vi "créer code EMBALLAGE_PAGO_V2.0.vi"(0 "DIVISION":enum16{"FLATPROP", "MEDIC"}(ring), 1 "N° carton":u8=1, 2 "DATA cmde":T2={"n°article FAS"="12-216C-04521 EQIFIL 417mA 14.4ohm", "n° cmde FAS"="03838/08-01.07.01", "quantité cmde"="75", "ID LIG cmde"="966584", "n° cmde client"="CF-08-0253/2", "nom client"="EMS Electro Medical System", "n° article client"="EL-360", "indice revision client"="03", "société de facturation"="Fas medic", "langue a utiliser"="FR"}, 5 "article":string="12-216C-04521 EQIFIL 417mA 14.4ohm", 7 "Nb pièces par carton":u8=25, 9 "Tableau n° valves":string[](array[string])=["112105740008010001", "112105740008010002", "112105740008010003", "112105740008010004", "112105740008010005", "112105740008010006", "112105740008010007", "112105740008010008", "112105740008010009", "112105740008010010", "112105740008010011", "112105740008010012", "112105740008010013", "112105740008010014", "112105740008010015", "112105740008010016", "112105740008010017", "112105740008010018", "112105740008010019", "112105740008010020", "112105740008010022", "112105740008010030", "112105740008010099", "112105740008020006", "112105740008020066"], 11 "error in (no error)":errorcluster caption="entrée d'erreur (pas d'erreur)", 12 "Tableau \nlots OUT":string[][](array[string]), 13 "Paramètres Produit (PP)":T1={"Numéro T121"="", "Créateur"="", "Date de création"="", "Date de modification"="", "indice produit"="", "Code Barre fixe"="", "Affiche n° Client [Oui/Non]"="", "Fichier PTV"="", "Nbr de valves / Cartons"="", "Mélange des lots posiible [Oui/Non] "="", "Affiche code barre client [Oui/Non]"="Non", "Fichier PP valve sur embase"="", "Valve Direct/Compensée [D/C]"="D"} caption="Paramètres produit", 14 "affiche code bar client":string="non") -> (6 "chaine  à écrire":string="ZB\nUS\nq600\nD7\nN\nR150,20\nI8,12,001\rA0,40,0,2,1,1,N,\"Carton : 1/2\"\rA0,85,0,2,1,1,N,\"Nb de valves : 25\"\rA0,130,0,2,1,1,N,\"Nø valves :\"\rA144,130,0,1,1,1,N,\"04235698, 05050505, 06060606, 06125478\"\rA144,146,0,1,1,1,N,\"06235511, 07070707, 08023326, 08080808\"\rA144,162,0,1,1,1,N,\"08080808, 08090909, 08110030, 08112347\"\rA144,178,0,1,1,1,N,\"08120003, 08120004, 08120025, 08121114\"\rA144,194,0,1,1,1,N,\"08123625, 08141254, 08152365, 08235644\"\rA144,210,0,1,1,1,N,\"08336251, 08452145, 08521456, 09040006\"\rA144,226,0,1,1,1,N,\"09090909\"\rB64,260,0,1,1,20,56,N,\"12-216C-04520 EQIFIL 104mA 36ohm\"\rA58,324,0,3,1,1,N,\"12...", 15 "error out":errorcluster caption="sortie d'erreur")   [LabVIEW 2020]
uses:
  Flatprop/Flatprop - Standard/XML/Control/PP Param_3.ctl
panel:
  out "n° cmde client":string="1/1"
  out "Destinataire":string="1/1"
  out "n° commande FAS":string="03838/08-07.01.01"
  out "n° valves 9-12":string
  out "Ref client":string="EL-360 "
  out "nom sous code bar client":string="EL-360  03 08010802 7"
  out "n° valves 46-50":string
  out "n° valves 41-45":string
  out "n° valves 36-40":string
  out "n° valves 25-28":string
  out "n° valves 21-24":string
  out "n° valves 17-20":string
  out "n° valves 13-16":string
  out "n° valves 5-8":string="08020006, 08020066"
  out "n° valves 1-4":string="08010003, 08010006, 08010009, 08010022, 08010099"
  out "Quantité":string="7/100"
  out "carton":string="1/1"
  out "nom valve FAS":string="12-216C-04520 EQIFIL 104mA 36ohm"
  # "Destinataire:"
  # "N°commande :"
  # "Quantité:"
  # "Votre ref.:"
  # "N° valves :\n(P/N)"
  # "FASmedic s.a.\nZone industrielle\nCH-1607 Palézieux-Gare\nTél.+41(0)21 907 79 71\nwww.fasmedic.com"
  # "N°article FAS:"
  # "N°commande FAS:"
  # "Carton :"
  # "etiquette"
  # "(Lien interchangeable)"
  # "emballage"
  # "emballage"
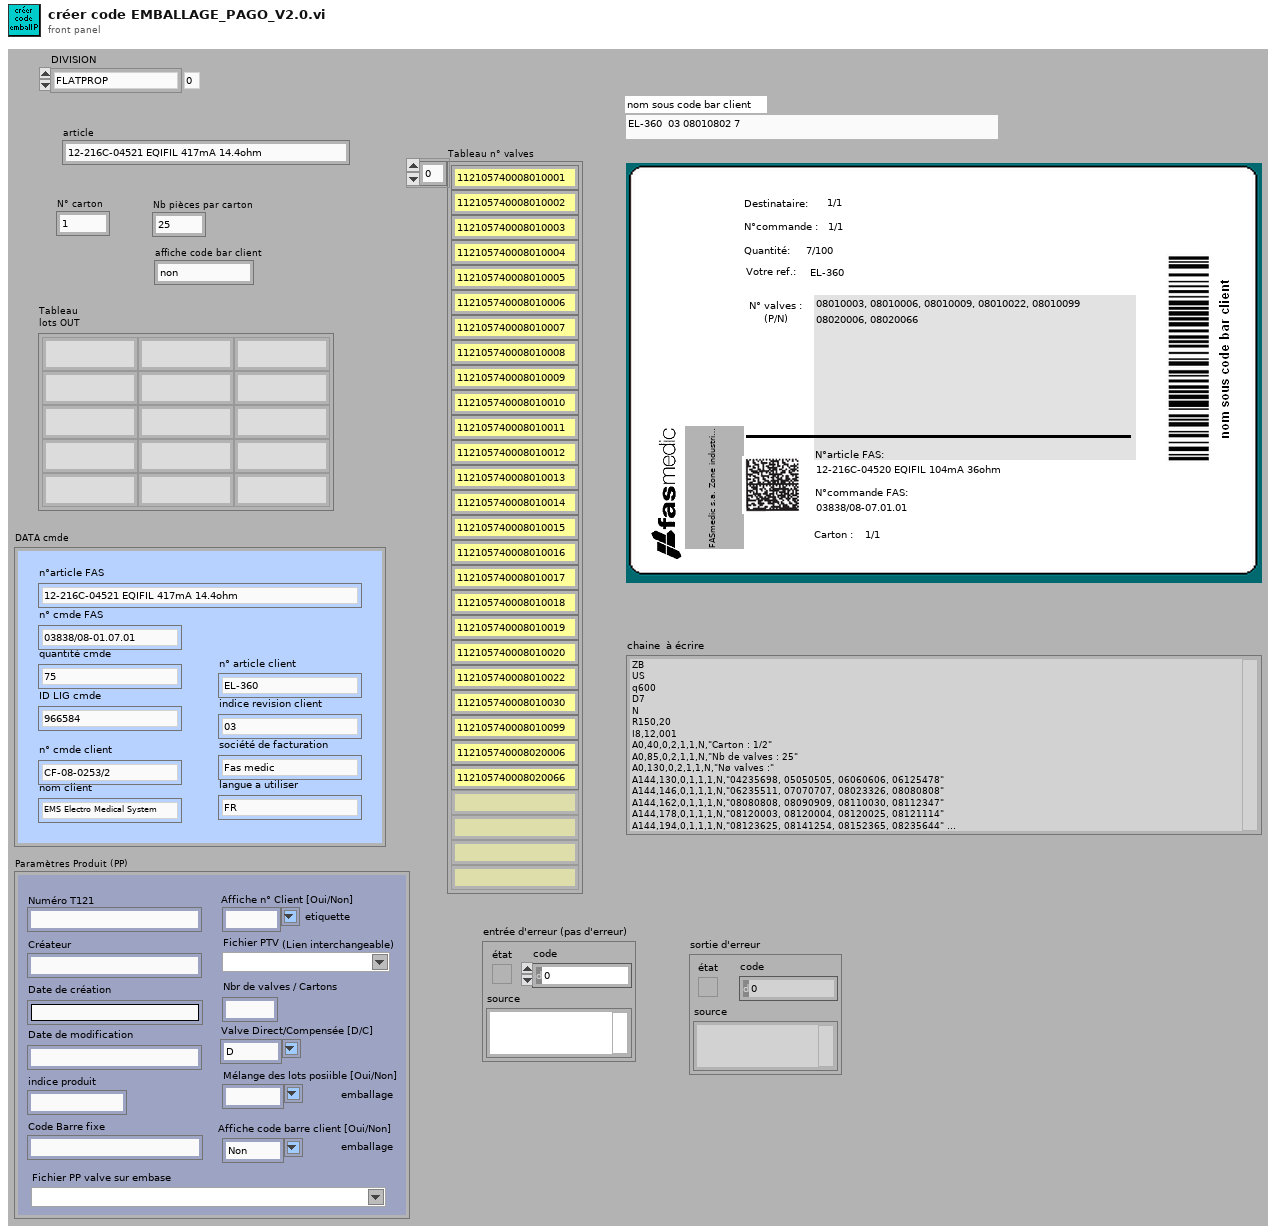
[diagram p1: front panel]
types:
  T1 = typedef "PP Param_3.ctl" = cluster{"Numéro T121":string, "Créateur":string, "Date de création":string, "Date de modification":string, "indice produit":string, "Code Barre fixe":string, "Affiche n° Client [Oui/Non]":string, "Fichier PTV":string, "Nbr de valves / Cartons":string, "Mélange des lots posiible [Oui/Non] ":string, "Affiche code barre client [Oui/Non]":string, "Fichier PP valve sur embase":string, "Valve Direct/Compensée [D/C]":string}
  T2 = typedef "DATA commande.ctl" = cluster{"n°article FAS":string, "n° cmde FAS":string, "quantité cmde":string, "ID LIG cmde":string, "n° cmde client":string, "nom client":string, "n° article client":string, "indice revision client":string, "société de facturation":string, "langue a utiliser":string}
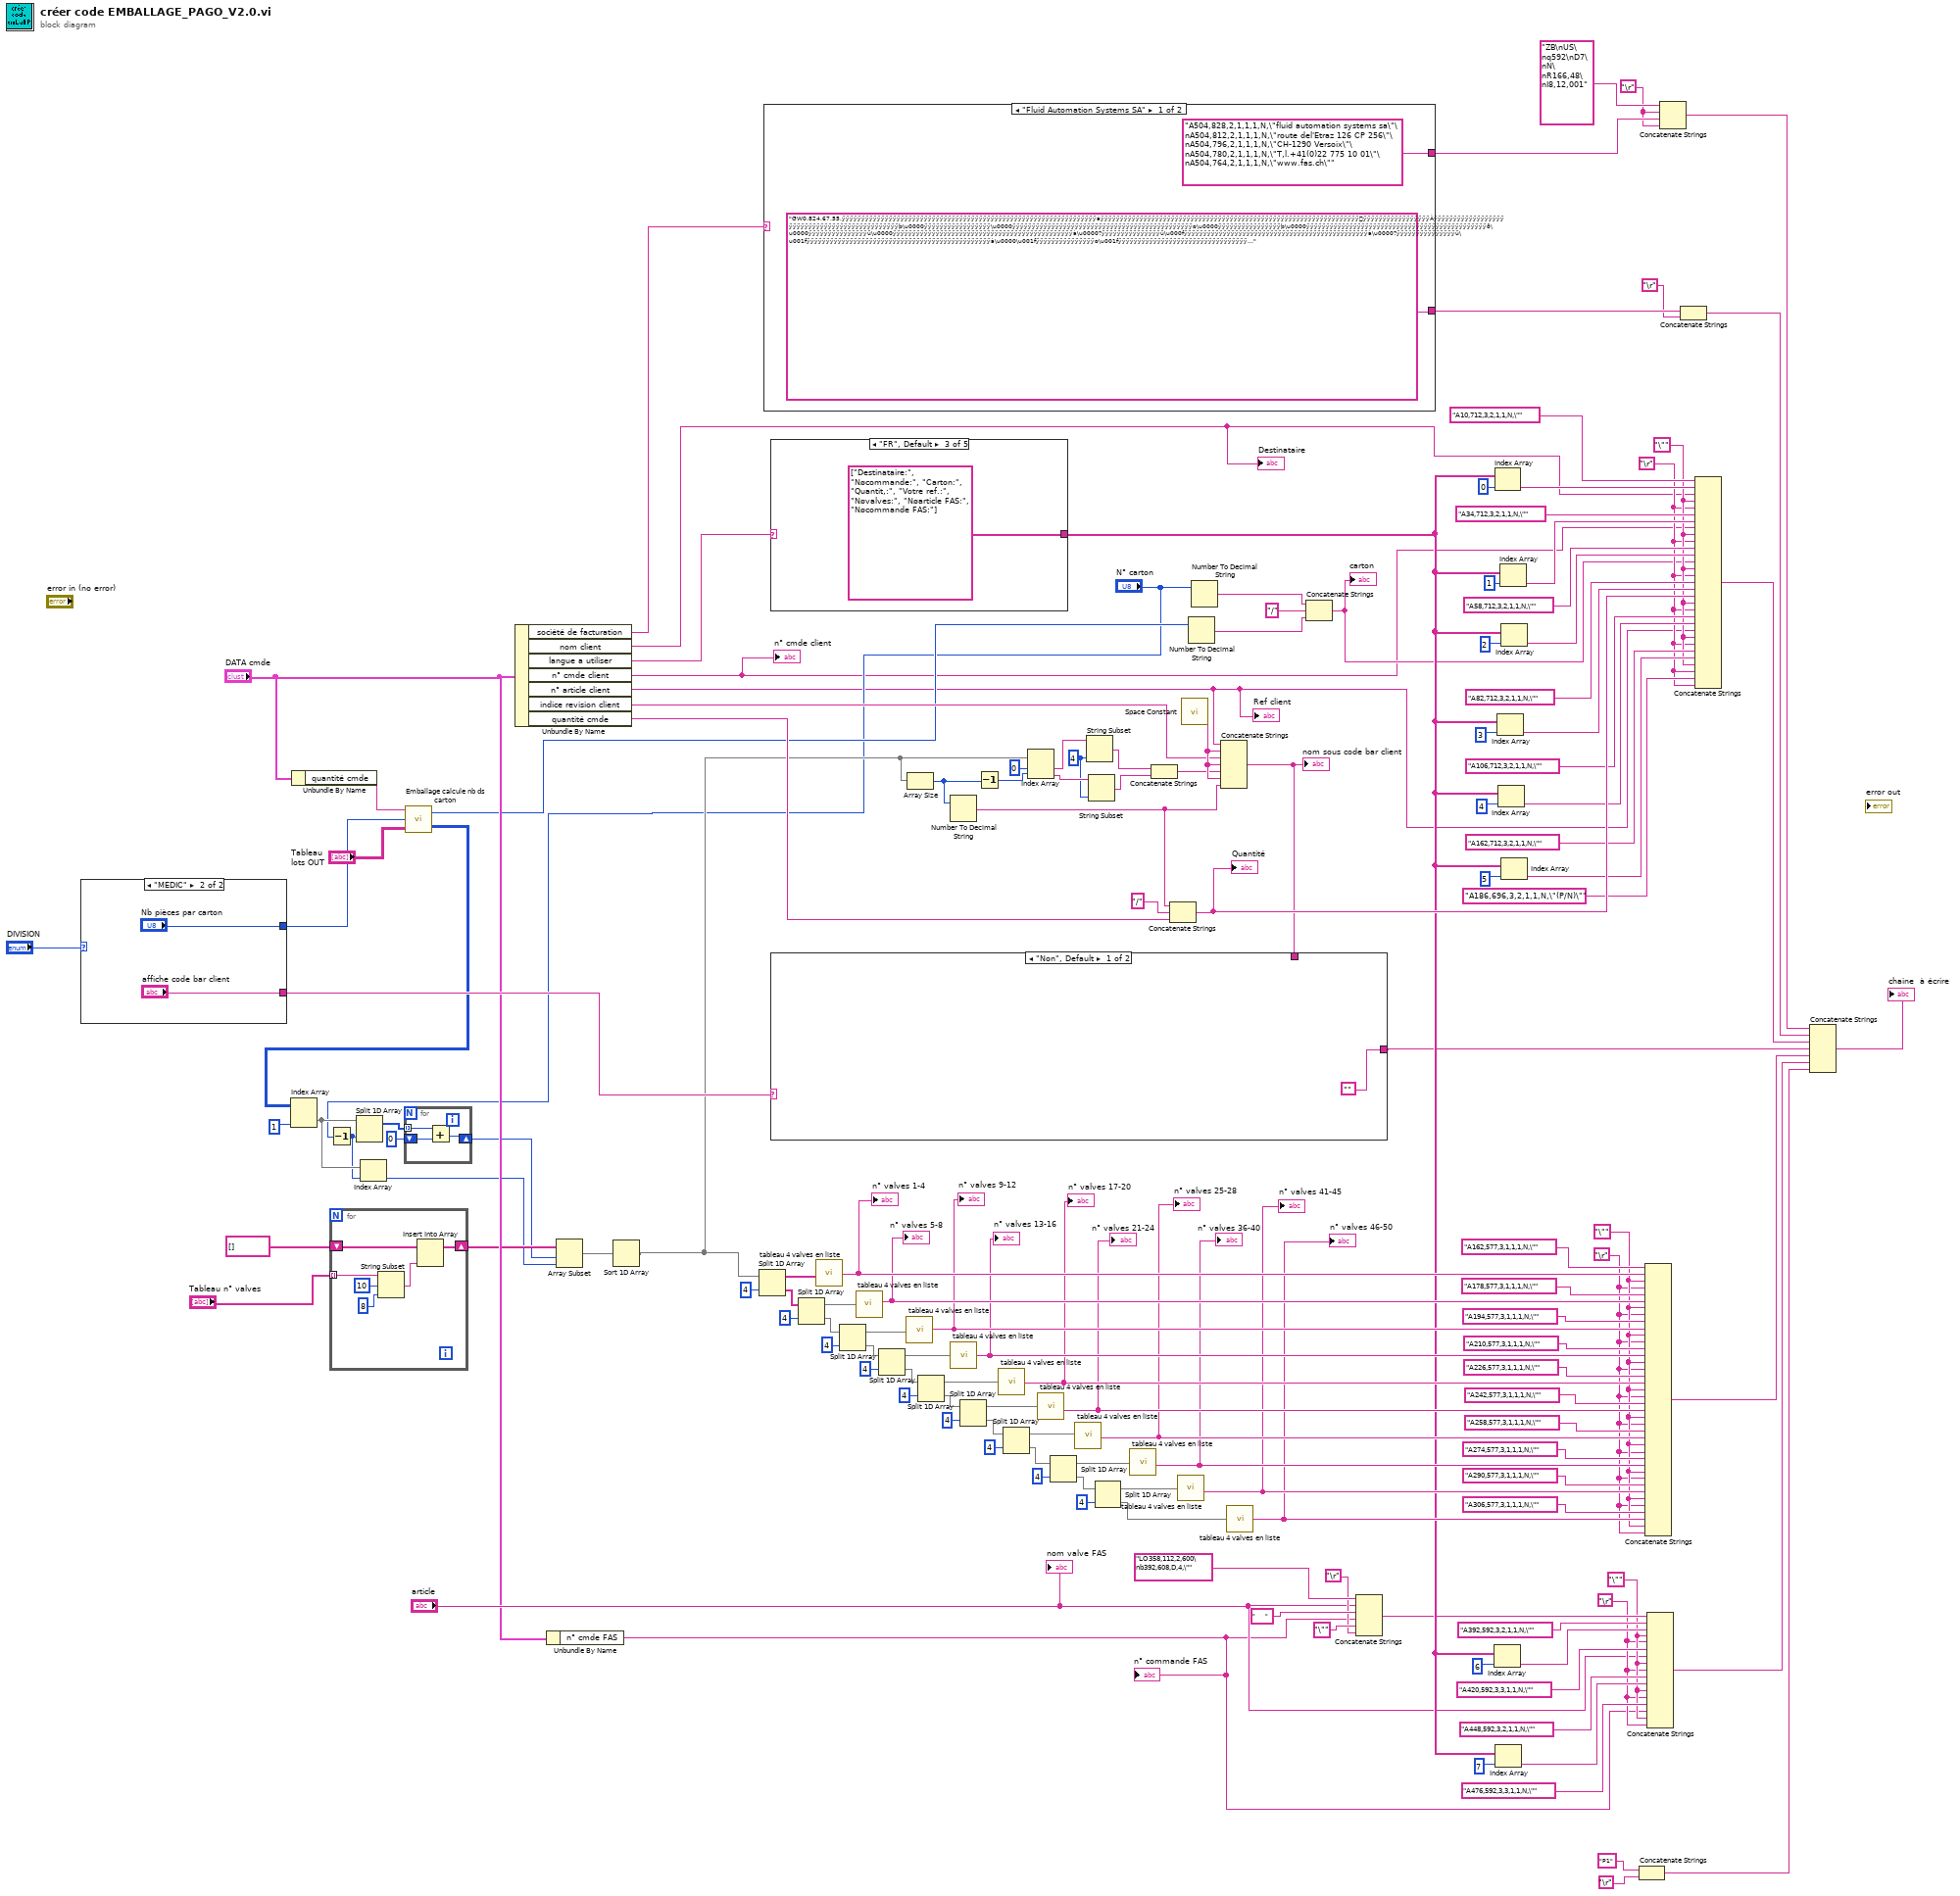
[diagram p0: block diagram]
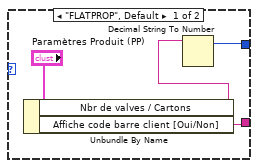
[diagram p2: hidden frame]
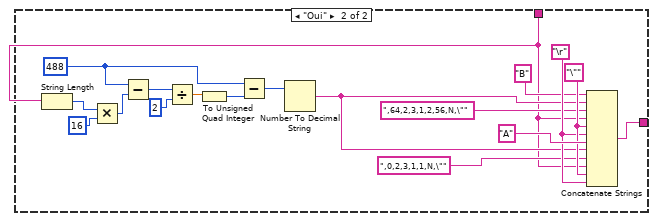
[diagram p3: hidden frame]
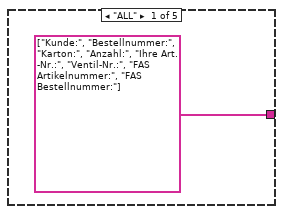
[diagram p4: hidden frame]
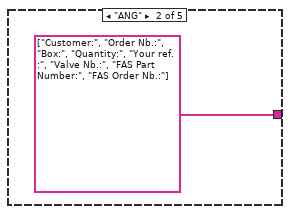
[diagram p5: hidden frame]
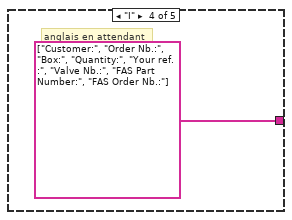
[diagram p6: hidden frame]
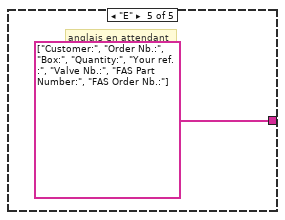
[diagram p7: hidden frame]
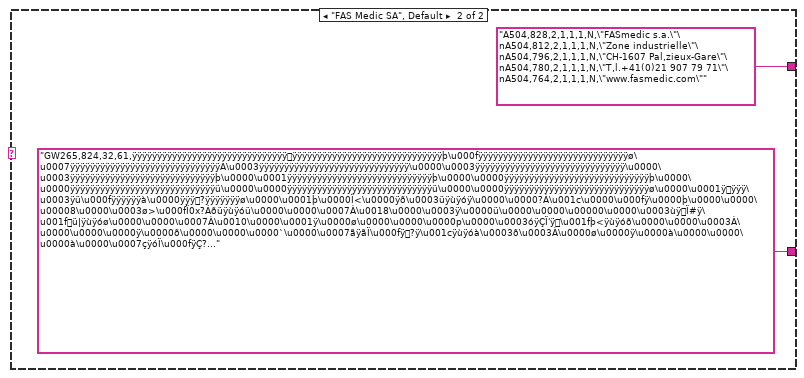
[diagram p8: hidden frame]
diagram:
  w47 = "\r"
  w48 = "\""
  w64 = "\""
  w63 = "\r"
  w87 = "\""
  w85 = "\r"
  w107 = "\r"
  w116 = 4 ("longueur (reste)")
  n1 = case shown="\"MEDIC\"" "DIVISION" {
    tunnel: [w149 "affiche code bar client"] -> w28
    tunnel: [w151 "Nb pièces par carton"] -> w25
    frame "FLATPROP", Default {
      n2 = Unbundle By Name("Paramètres Produit (PP)") -> ("Nbr de valves / Cartons"=w150:string, "Affiche code barre client [Oui/Non]"=w149:string)
      n3 = Decimal String To Number(string=w150) -> (offset past number=w151:i32)  [unwired: 2 in, 1 out]
    }
    frame "MEDIC" {
    }
  }
  n4 = Unbundle By Name("DATA cmde") -> ("quantité cmde"=w23:string)
  n5 = Decrement(x="N° carton") -> (x-1=w12:u8)
  n6 = for {
    tunnel: "Tableau n° valves" -> [w160] mode=indexing
    shift-right: [w157] -> w18
    shift-left: string[] [] -> [w156]
    n7 = String Subset(string=w160, offset (0)=10, length (rest)=8 ("longueur (reste)")) -> (substring=w158:string)
    n8 = Insert Into Array(array=w156, new element=w158) -> (w157:string[])  [unwired: 1 in]
  }
  n9 = call "Emballage calcule nb ds carton.vi"("Tableau \nlots OUT"="Tableau \nlots OUT", 3:w25, "Quantité de la cmde"=w23) -> ("Tab n° carton - nb ds carton"=w7:i32[][], "Nb total cartons"=w6:i32)
  n10 = Index Array(array=w7, index (col)=1 ("indice désactivé (col)")) -> (element=w13:i32[])  [unwired: 1 in]
  n11 = Split 1D Array(array=w13, index=w12) -> (first subarray=w15:i32[])  [unwired: 1 out]
  n12 = Index Array(array=w13, index=w12) -> (element=w11:i32)
  n13 = for {
    tunnel: w15 -> [w163] mode=indexing
    shift-right: [w161] -> w14
    shift-left: 0 -> [w162]
    n14 = Add(x=w163, y=w162) -> (x+y=w161:i32)
  }
  n15 = Unbundle By Name("DATA cmde") -> ("société de facturation"=w31:string, "nom client"=w2:string, "langue a utiliser"=w32:string, "n° cmde client"=w1:string, "indice revision client"=w30:string, "quantité cmde"=w29:string)  [unwired: 1 out]
  "Ref client" <- w1
  "Destinataire" <- w2
  "n° cmde client" <- w1
  n16 = Unbundle By Name("DATA cmde") -> ("n° cmde FAS"=w27:string)
  "n° commande FAS" <- w27
  n17 = Array Subset(array=w18, index=w14, length=w11) -> (w17:string[])
  n18 = Sort 1D Array(array=w17) -> (sorted array=w9:string[])
  n19 = Split 1D Array(array=w9, index=4 ("indice")) -> (first subarray=w139:string[], second subarray=w146:string[])
  n20 = case shown="\"Fluid Automation Systems SA\"" w31 {
    tunnel: ["GW0,824,67,55,ÿÿÿÿÿÿÿÿÿÿÿÿÿÿÿÿÿÿÿÿÿÿÿÿÿÿÿÿÿÿÿÿÿÿÿÿÿÿÿÿÿÿÿÿÿÿÿÿÿÿÿÿÿÿÿÿÿÿÿÿÿÿÿÿÿáÿÿÿÿÿÿÿÿÿÿÿÿÿÿÿÿÿÿÿÿÿÿÿÿÿÿÿÿÿÿÿÿÿÿÿÿÿÿÿÿÿÿÿÿÿÿÿÿÿÿÿÿÿÿÿÿÿÿÿÿÿÿÿÿÿÿÿÿÿÿÿÿÿÿÿÿÿÿÿÿÿÿÿÀÿÿÿÿÿÿÿÿÿÿÿÿÿÿÿÿÿÿÿÿÿÿÿÿÿÿÿÿÿÿÿÿÿÿÿÿÿÿÿÿÿÿÿÿÿÿþ\u0000ÿÿÿÿÿÿÿÿÿÿÿÿÿÿÿÿÿ\u0000ÿÿÿÿÿÿÿÿÿÿÿÿÿÿÿÿÿÿÿÿÿÿÿÿÿÿÿÿÿÿÿÿÿÿÿÿÿÿÿÿÿÿÿÿÿÿø\u0000ÿÿÿÿÿÿÿÿÿÿÿÿÿÿÿÿþ\u0000ÿÿÿÿÿÿÿÿÿÿÿÿÿÿÿÿÿÿÿÿÿÿÿÿÿÿÿÿÿÿÿÿÿÿÿÿÿÿÿÿÿÿÿÿÿÿð\u0000ÿÿÿÿÿÿÿÿÿÿÿÿÿÿÿü\u0000ÿÿÿÿÿÿÿÿÿÿÿÿÿÿÿÿÿÿÿÿÿÿÿÿÿÿÿÿÿÿÿÿÿÿÿÿÿÿÿÿÿÿÿÿÿÿà\u0000?ÿÿÿÿÿÿÿÿÿÿÿÿÿÿÿü\u000fÿÿÿÿÿÿÿÿÿÿÿÿÿÿÿÿÿÿÿÿÿÿÿÿÿÿÿÿÿÿÿÿÿÿÿÿÿÿÿÿÿÿÿÿÿÿÿà\u0000?ÿÿÿÿÿÿÿÿÿÿÿÿÿÿÿü\u001fÿÿÿÿÿÿÿÿÿÿÿÿÿÿÿÿÿÿÿÿÿÿÿÿÿÿÿÿÿÿÿÿÿÿÿÿÿÿÿÿÿÿÿÿÿÿÿà\u0000\u001fÿÿÿÿÿÿÿÿÿÿÿÿÿÿÿø\u001fÿÿÿÿÿÿÿÿÿÿÿÿÿÿÿÿÿÿÿÿÿÿÿÿÿÿÿÿÿÿÿÿÿ..." "GW265,824,32,61,ÿÿÿÿÿÿÿÿÿÿÿÿÿÿÿÿÿÿÿÿÿÿÿÿÿÿÿÿÿÿÿÿÿÿÿÿÿÿÿÿÿÿÿÿÿÿÿÿÿÿÿÿÿÿÿÿÿÿÿÿÿþ\u000fÿÿÿÿÿÿÿÿÿÿÿÿÿÿÿÿÿÿÿÿÿÿÿÿÿÿÿÿÿÿø\u0007ÿÿÿÿÿÿÿÿÿÿÿÿÿÿÿÿÿÿÿÿÿÿÿÿÿÿÿÿÿÿÀ\u0003ÿÿÿÿÿÿÿÿÿÿÿÿÿÿÿÿÿÿÿÿÿÿÿÿÿÿÿÿÿÿ\u0000\u0003ÿÿÿÿÿÿÿÿÿÿÿÿÿÿÿÿÿÿÿÿÿÿÿÿÿÿÿÿÿÿ\u0000\u0003ÿÿÿÿÿÿÿÿÿÿÿÿÿÿÿÿÿÿÿÿÿÿÿÿÿÿÿÿÿþ\u0000\u0001ÿÿÿÿÿÿÿÿÿÿÿÿÿÿÿÿÿÿÿÿÿÿÿÿÿÿÿÿÿþ\u0000\u0000ÿÿÿÿÿÿÿÿÿÿÿÿÿÿÿÿÿÿÿÿÿÿÿÿÿÿÿÿÿþ\u0000\u0000ÿÿÿÿÿÿÿÿÿÿÿÿÿÿÿÿÿÿÿÿÿÿÿÿÿÿÿÿÿü\u0000\u0000ÿÿÿÿÿÿÿÿÿÿÿÿÿÿÿÿÿÿÿÿÿÿÿÿÿÿÿÿÿü\u0000\u0000ÿÿÿÿÿÿÿÿÿÿÿÿÿÿÿÿÿÿÿÿÿÿÿÿÿÿÿÿÿø\u0000\u0001ÿÿÿÿ\u0003ÿü\u000fÿÿÿÿÿÿà\u0000ÿÿÿ?ÿÿÿÿÿÿÿø\u0000\u0001þ\u0000Ï<\u0000ÿð\u0003üÿùÿóÿ\u0000\u0000?À\u001c\u0000\u000fÿ\u0000þ\u0000\u0000\u00008\u0000\u0003ø>\u000fÏ0x?Áðüÿùÿóü\u0000\u0000\u0007À\u0018\u0000\u0003ÿ\u0000ü\u0000\u0000\u00000\u0000\u0003ùÿÏ#ÿ\u001fü|ÿùÿóø\u0000\u0000\u0007À\u0010\u0000\u0001ÿ\u0000ø\u0000\u0000\u0000p\u0000\u0003óÿÇÏ'ÿ\u001fþ<ÿùÿóð\u0000\u0000\u0003À\u0000\u0000\u0000ÿ\u0000ð\u0000\u0000\u0000`\u0000\u0007ãÿãÏ\u000fÿ?ÿ\u001cÿùÿóà\u0003ð\u0003À\u0000ø\u0000ÿ\u0000à\u0000\u0000\u0000à\u0000\u0007çÿóÏ\u000fÿÇ?..."] -> w44
    tunnel: ["A504,828,2,1,1,1,N,\"fluid automation systems sa\"\nA504,812,2,1,1,1,N,\"route del'Etraz 126 CP 256\"\nA504,796,2,1,1,1,N,\"CH-1290 Versoix\"\nA504,780,2,1,1,1,N,\"T‚l.+41(0)22 775 10 01\"\nA504,764,2,1,1,1,N,\"www.fas.ch\"" "A504,828,2,1,1,1,N,\"FASmedic s.a.\"\nA504,812,2,1,1,1,N,\"Zone industrielle\"\nA504,796,2,1,1,1,N,\"CH-1607 Pal‚zieux-Gare\"\nA504,780,2,1,1,1,N,\"T‚l.+41(0)21 907 79 71\"\nA504,764,2,1,1,1,N,\"www.fasmedic.com\""] -> w108
    frame "Fluid Automation Systems SA" {
    }
    frame "FAS Medic SA", Default {
    }
  }
  n21 = case shown="\"FR\", Default" w32 {
    tunnel: [string[] ["Kunde:", "Bestellnummer:", "Karton:", "Anzahl:", "Ihre Art.-Nr.:", "Ventil-Nr.:", "FAS Artikelnummer:", "FAS Bestellnummer:"] string[] ["Customer:", "Order Nb.:", "Box:", "Quantity:", "Your ref.:", "Valve Nb.:", "FAS Part Number:", "FAS Order Nb.:"] string[] ["Destinataire:", "Nøcommande:", "Carton:", "Quantit‚:", "Votre ref.:", "Nøvalves:", "Nøarticle FAS:", "Nøcommande FAS:"] string[] ["Customer:", "Order Nb.:", "Box:", "Quantity:", "Your ref.:", "Valve Nb.:", "FAS Part Number:", "FAS Order Nb.:"] string[] ["Customer:", "Order Nb.:", "Box:", "Quantity:", "Your ref.:", "Valve Nb.:", "FAS Part Number:", "FAS Order Nb.:"]] -> w57
    frame "ALL" {
    }
    frame "ANG" {
    }
    frame "FR", Default {
    }
    frame "I" {
      # "anglais en attendant"
    }
    frame "E" {
      # "anglais en attendant"
    }
  }
  n22 = Split 1D Array(array=w146, index=4 ("indice")) -> (first subarray=w138:string[], second subarray=w144:string[])
  n23 = call "tableau 4 valves en liste.vi"("Tableau de 4 valves"=w139) -> ("Chaîne de 5 valves"=w83:string)
  "n° valves 1-4" <- w83
  n24 = Split 1D Array(array=w144, index=4 ("indice")) -> (first subarray=w137:string[], second subarray=w142:string[])
  n25 = call "tableau 4 valves en liste.vi"("Tableau de 4 valves"=w138) -> ("Chaîne de 5 valves"=w81:string)
  "n° valves 5-8" <- w81
  n26 = Split 1D Array(array=w142, index=4 ("indice")) -> (first subarray=w136:string[], second subarray=w140:string[])
  n27 = call "tableau 4 valves en liste.vi"("Tableau de 4 valves"=w137) -> ("Chaîne de 5 valves"=w80:string)
  "n° valves 9-12" <- w80
  n28 = Array Size(array=w9) -> (size(s)=w112:i32)
  n29 = Split 1D Array(array=w140, index=4 ("indice")) -> (first subarray=w135:string[], second subarray=w133:string[])
  n30 = Number To Decimal String(number=w112) -> (decimal integer string=w110:string)  [unwired: 1 in]
  n31 = call "tableau 4 valves en liste.vi"("Tableau de 4 valves"=w136) -> ("Chaîne de 5 valves"=w77:string)
  "n° valves 13-16" <- w77
  n32 = Split 1D Array(array=w133, index=4 ("indice")) -> (first subarray=w132:string[], second subarray=w130:string[])
  n33 = Decrement(x=w112) -> (x-1=w113:i32)
  n34 = call "tableau 4 valves en liste.vi"("Tableau de 4 valves"=w135) -> ("Chaîne de 5 valves"=w76:string)
  "n° valves 17-20" <- w76
  n35 = Split 1D Array(array=w130, index=4 ("indice")) -> (first subarray=w129:string[], second subarray=w127:string[])
  n36 = Index Array(array=w9, index #1=0 ("indice"), index #2=w113) -> (element #1=w118:string, element #2=w117:string)
  n37 = call "tableau 4 valves en liste.vi"("Tableau de 4 valves"=w132) -> ("Chaîne de 5 valves"=w73:string)
  "n° valves 21-24" <- w73
  n38 = Split 1D Array(array=w127, index=4 ("indice")) -> (first subarray=w126:string[], second subarray=w124:string[])
  n39 = call "tableau 4 valves en liste.vi"("Tableau de 4 valves"=w129) -> ("Chaîne de 5 valves"=w71:string)
  "n° valves 25-28" <- w71
  n40 = String Subset(string=w118, length (rest)=w116) -> (substring=w115:string)  [unwired: 1 in]
  n41 = String Subset(string=w117, length (rest)=w116) -> (substring=w114:string)  [unwired: 1 in]
  n42 = Split 1D Array(array=w124, index=4 ("indice")) -> (first subarray=w123:string[], second subarray=w122:string[])
  n43 = call "tableau 4 valves en liste.vi"("Tableau de 4 valves"=w126) -> ("Chaîne de 5 valves"=w69:string)
  "n° valves 36-40" <- w69
  n44 = Concatenate Strings(w115, w114) -> (w119:string)
  n45 = Concatenate Strings(w110, "/" ("chaîne"), w29) -> (w94:string)
  "Quantité" <- w94
  n46 = call "tableau 4 valves en liste.vi"("Tableau de 4 valves"=w123) -> ("Chaîne de 5 valves"=w67:string)
  "n° valves 41-45" <- w67
  n47 = call <vilib>:"Space Constant.vi"() -> ("String"=w120:string)
  n48 = Number To Decimal String(number=w6) -> (decimal integer string=w20:string)  [unwired: 1 in]
  n49 = Number To Decimal String(number="N° carton") -> (decimal integer string=w22:string)  [unwired: 1 in]
  n50 = Concatenate Strings(w1, w120, w30, w120, w119, w120, w110) -> (w35:string)
  "nom sous code bar client" <- w35
  n51 = case shown="\"Non\", Default" w28 {
    tunnel: w35 -> [_ w174]
    tunnel: ["" w188] -> w34
    frame "Non", Default {
    }
    frame "Oui" {
      w182 = 488
      w190 = "\""
      w189 = "\r"
      n52 = String Length(string=w174) -> (length=w187:i32)
      n53 = Multiply(x=w187, y=16) -> (x*y=w185:i32)
      n54 = Subtract(x=w182, y=w185) -> (x-y=w184:i32)
      n55 = Divide(x=w184, y=2) -> (x/y=w181:dbl)
      n56 = To Unsigned Quad Integer(1:w181) -> (0:w180:u64)
      n57 = Subtract(x=w182, y=w180) -> (x-y=w179:u64)
      n58 = Number To Decimal String(number=w179) -> (decimal integer string=w175:string)  [unwired: 1 in]
      n59 = Concatenate Strings("B", w175, ",64,2,3,1,2,56,N,\"", w174, w190, w189, "A", w175, ",0,2,3,1,1,N,\"", w174, w190, w189) -> (w188:string)
    }
  }
  n60 = call "tableau 4 valves en liste.vi"("Tableau de 4 valves"=w122) -> ("Chaîne de 5 valves"=w65:string)
  "n° valves 46-50" <- w65
  n61 = Concatenate Strings(w22, "/", w20) -> (w4:string)
  "carton" <- w4
  n62 = Concatenate Strings("LO358,112,2,600\nb392,608,D,4,\"", "article", "     ", w27, "\"", "\r") -> (w55:string)
  n63 = Index Array(array=w57, index=6 ("indice")) -> (element=w53:string)
  n64 = Index Array(array=w57, index=0 ("indice")) -> (element=w104:string)
  n65 = Index Array(array=w57, index=7 ("indice")) -> (element=w50:string)
  n66 = Index Array(array=w57, index=3 ("indice")) -> (element=w95:string)
  n67 = Index Array(array=w57, index=4 ("indice")) -> (element=w92:string)
  n68 = Index Array(array=w57, index=1 ("indice")) -> (element=w101:string)
  n69 = Index Array(array=w57, index=2 ("indice")) -> (element=w98:string)
  n70 = Index Array(array=w57, index=5 ("indice")) -> (element=w88:string)
  n71 = Concatenate Strings("P1", "\r") -> (w37:string)
  n72 = Concatenate Strings("A162,577,3,1,1,1,N,\"", w83, w64, w63, "A178,577,3,1,1,1,N,\"", w81, w64, w63, "A194,577,3,1,1,1,N,\"", w80, w64, w63, "A210,577,3,1,1,1,N,\"", w77, w64, w63, "A226,577,3,1,1,1,N,\"", w76, w64, w63, "A242,577,3,1,1,1,N,\"", w73, w64, w63, "A258,577,3,1,1,1,N,\"", w71, w64, w63, "A274,577,3,1,1,1,N,\"", w69, w64, w63, "A290,577,3,1,1,1,N,\"", w67, w64, w63, "A306,577,3,1,1,1,N,\"", w65, w64, w63) -> (w39:string)
  n73 = Concatenate Strings(w55, "A392,592,3,2,1,1,N,\"", w53, w48, w47, "A420,592,3,3,1,1,N,\"", "article", w48, w47, "A448,592,3,2,1,1,N,\"", w50, w48, w47, "A476,592,3,3,1,1,N,\"", w27, w48, w47) -> (w38:string)
  n74 = Concatenate Strings("ZB\nUS\nq592\nD7\nN\nR166,48\nI8,12,001", w107, w108, w107) -> (w42:string)
  n75 = Concatenate Strings(w44, "\r") -> (w41:string)
  n76 = Concatenate Strings("A10,712,3,2,1,1,N,\"", w104, w2, w87, w85, "A34,712,3,2,1,1,N,\"", w101, w1, w87, w85, "A58,712,3,2,1,1,N,\"", w98, w4, w87, w85, "A82,712,3,2,1,1,N,\"", w95, w94, w87, w85, "A106,712,3,2,1,1,N,\"", w92, w1, w87, w85, "A162,712,3,2,1,1,N,\"", w88, w87, w85, "A186,696,3,2,1,1,N,\"(P/N)\"", w85) -> (w40:string)
  n77 = Concatenate Strings(w42, w41, w40, w34, w39, w38, w37) -> (→"chaine  à écrire":string)
  "nom valve FAS" <- "article"
